vi "Calc Next Rate or Stop.vi"(6 "Target Rate":dbl, 7 "Converge Target":dbl, 8 "error in (no error)":errorcluster, 9 "Iteration":i32, 10 "Test Info In":T1, 11 "Possible Failure Modes":bool[](array[boolean])) -> (0 "error out":errorcluster, 1 "CurProg":dbl, 2 "Test Info Out":T1, 3 "Stop?":bool, 4 "Next Rate":dbl)   [LabVIEW 2011]
uses:
  Test Info.ctl
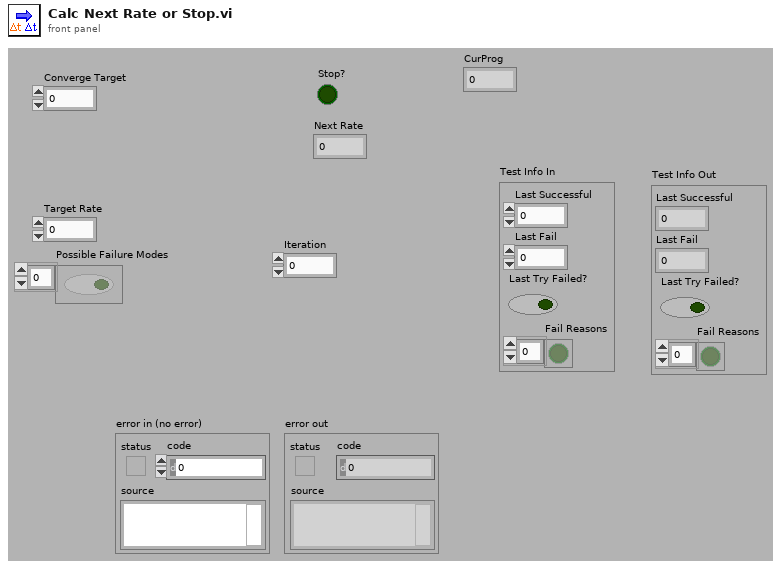
[diagram p1: front panel]
types:
  T1 = typedef "Test Info.ctl" = cluster{"Last Successful":dbl, "Last Fail":dbl, "Last Try Failed?":bool, "Fail Reasons":bool[]}
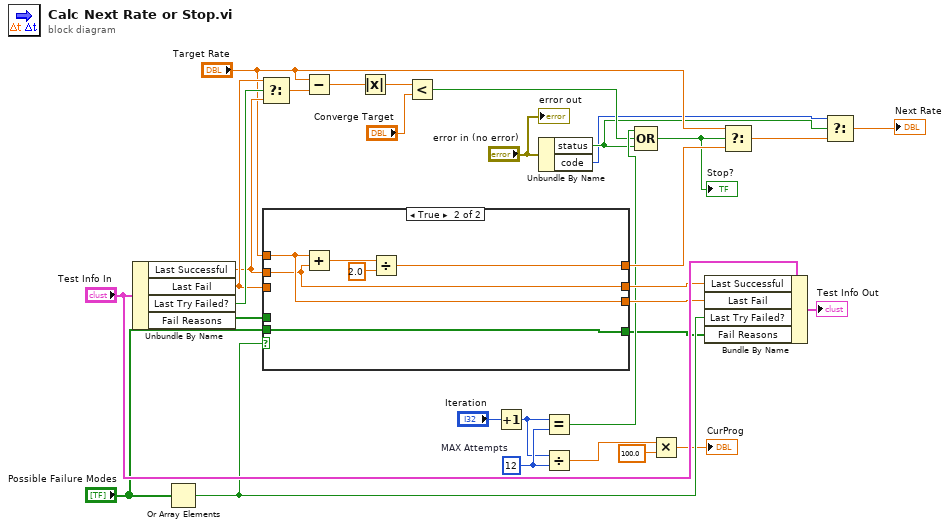
[diagram p0: block diagram]
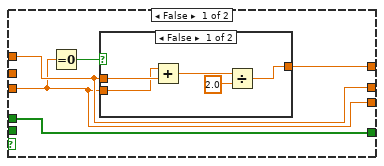
[diagram p2: hidden frame]
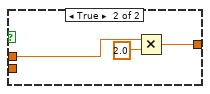
[diagram p3: hidden frame]
diagram:
  w15 = 12  # MAX Attempts
  n1 = Unbundle By Name("Test Info In") -> ("Last Successful"=w22:dbl, "Last Fail"=w23:dbl, "Last Try Failed?"=w24:bool, "Fail Reasons"=w3:bool[])
  n2 = Or Array Elements(Boolean array="Possible Failure Modes") -> (logical OR=w18:bool)
  n3 = Select(t=w23, s=w24, f=w22) -> (s? t:f=w21:dbl)
  n4 = case shown="True" w18 {
    tunnel: "Target Rate" -> [w34 w47]
    tunnel: w23 -> [w33 _]
    tunnel: w22 -> [_ w46]
    tunnel: [w36 w48] -> w19
    tunnel: [w33 w47] -> w26
    tunnel: [w34 w46] -> w25
    tunnel: [w32 w45] -> w4
    tunnel: w3 -> [w32 _]
    tunnel: "Possible Failure Modes" -> [_ w45]
    frame False {
      n5 = Equal To 0?(x=w33) -> (x = 0?=w35:bool)
      n6 = case shown="False" w35 {
        tunnel: w34 -> [w39 w43]
        tunnel: [w37 w42] -> w36
        tunnel: w33 -> [w38 _]
        frame False {
          n7 = Add(x=w38, y=w39) -> (x+y=w41:dbl)
          n8 = Divide(x=w41, y=2.0) -> (x/y=w37:dbl)
        }
        frame True {
          n9 = Multiply(x=w43, y=2.0) -> (x*y=w42:dbl)
        }
      }
    }
    frame True {
      n10 = Add(x=w47, y=w46) -> (x+y=w50:dbl)
      n11 = Divide(x=w50, y=2.0) -> (x/y=w48:dbl)
    }
  }
  n12 = Subtract(x="Target Rate", y=w21) -> (x-y=w31:dbl)
  n13 = Absolute Value(x=w31) -> (abs(x)=w30:dbl)
  n14 = Less?(x=w30, y="Converge Target") -> (x < y?=w9:bool)
  n15 = Increment(x="Iteration") -> (x+1=w1:i32)
  n16 = Unbundle By Name("error in (no error)") -> ("status"=w8:bool, "code"=w6:i32)
  n17 = Equal?(x=w1, y=w15) -> (x = y?=w10:bool)
  n18 = Divide(x=w1, y=w15) -> (x/y=w14:dbl)
  n19 = Compound Arithmetic op=OR(w10, w9, w8) -> (w17:bool)
  "Stop?" <- w17
  n20 = Multiply(x=w14, y=100.0) -> (x*y=→"CurProg":dbl)
  n21 = Bundle By Name(cluster="Test Info In", "Last Successful"=w25, "Last Fail"=w26, "Last Try Failed?"=w18, "Fail Reasons"=w4) -> (→"Test Info Out":T1)
  n22 = Select(t="Target Rate", s=w17, f=w19) -> (s? t:f=w7:dbl)
  n23 = Select(t=w6, s=w8, f=w7) -> (s? t:f=→"Next Rate":dbl)
  "error out" <- "error in (no error)"
